vi "UI_setPlayer.vi"(7 "action":enum16{"set refs", "set player", "next player"}(ring)=enum."next player", 8 "error in (no error)":errorcluster, 9 "player":enum16{"one", "two", "three"}(ring), 11 "LED refs":refnum<vi>[](array[refnum])) -> (0 "error out":errorcluster, 2 "Player":i32)   [LabVIEW 2020]
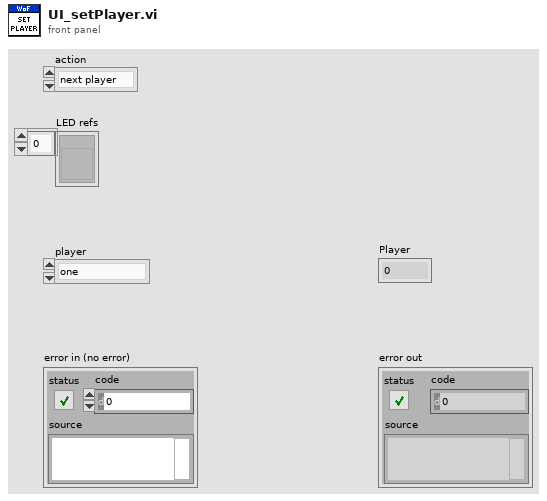
[diagram p1: front panel]
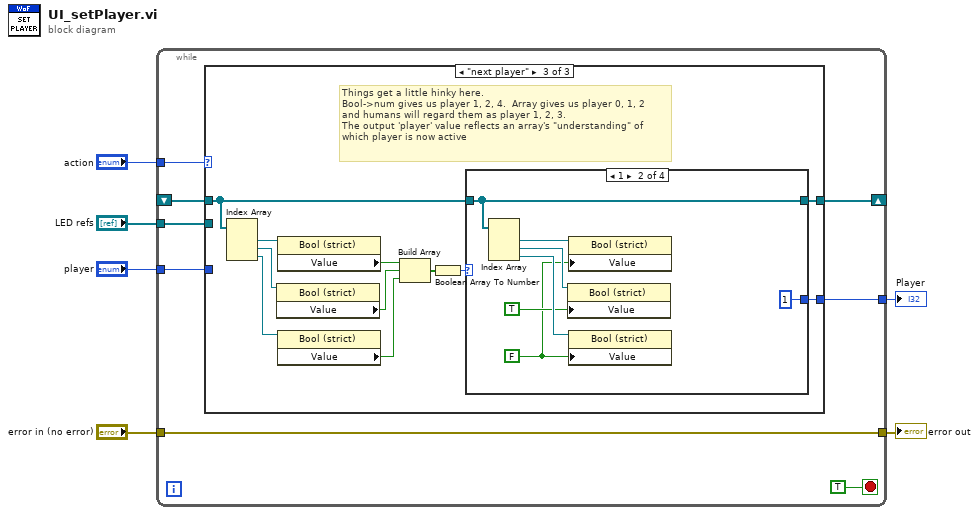
[diagram p0: block diagram]
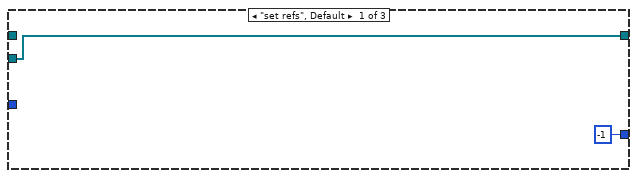
[diagram p2: hidden frame]
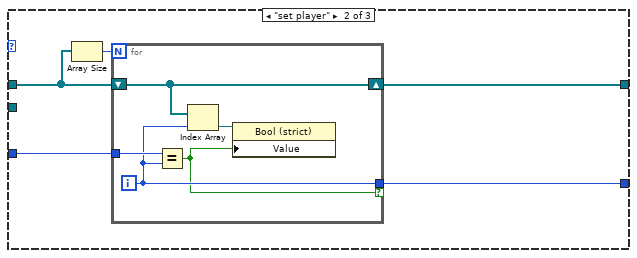
[diagram p3: hidden frame]
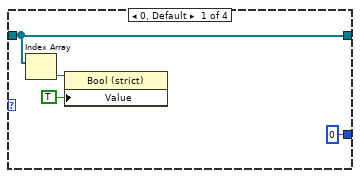
[diagram p4: hidden frame]
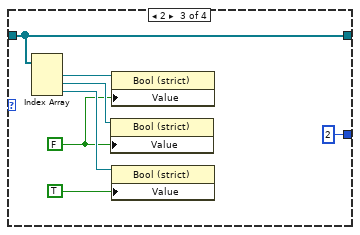
[diagram p5: hidden frame]
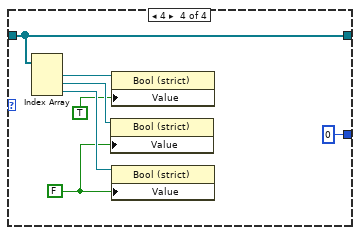
[diagram p6: hidden frame]
diagram:
  n1 = while {
    tunnel: "action" -> [w14]
    tunnel: "player" -> [w13]
    tunnel: "LED refs" -> [w11]
    shift-right: [w10] -> _
    shift-left: _ -> [w9]
    tunnel: [w8] -> w3
    tunnel: "error in (no error)" -> [w7]
    tunnel: [w7] -> w1
    stop <- TRUE stop-if-true
    n2 = case shown="\"next player\"" w14 {
      tunnel: w13 -> [_ w20 _]
      tunnel: w11 -> [w16 _ _]
      tunnel: [w16 w21 w28] -> w10
      tunnel: w9 -> [_ w18 w30]
      tunnel: [-1 w19 w27] -> w8
      frame "set refs", Default {
      }
      frame "set player" {
        n3 = Array Size(array=w18) -> (size(s)=w17:i32)
        n4 = for {
          N: w17 -> [_]
          shift-right: [w26] -> w21
          shift-left: w18 -> [w26]
          tunnel: w20 -> [w25]
          tunnel: [w24] -> w19 if=w22
          i -> [w24]
          n5 = Equal?(x=w25, y=w24) -> (x = y?=w22:bool)
          n6 = Index Array(array=w26, index=w24) -> (element=w23:refnum<vi>)
          n7 = property class="Bool (strict)"(reference=w23, "Value"=w22) -> ()  [unwired: 1 in, 2 out]
        }
      }
      frame "next player" {
        # "Things get a little hinky here.\nBool->num gives us player 1, 2, 4.  Array gives us player 0, 1, 2\nand humans will regard them as player 1, 2, 3.\nThe output 'player' value reflects an array's \"understanding\" of\nwhich player is now active"
        n8 = Index Array(array=w30) -> (element #1=w37:refnum<vi>, element #2=w36:refnum<vi>, element #3=w35:refnum<vi>)  [unwired: 3 in]
        n9 = property class="Bool (strict)"(reference=w36) -> ("Value"=w33:bool)  [unwired: 1 in, 2 out]
        n10 = property class="Bool (strict)"(reference=w37) -> ("Value"=w34:bool)  [unwired: 1 in, 2 out]
        n11 = property class="Bool (strict)"(reference=w35) -> ("Value"=w32:bool)  [unwired: 1 in, 2 out]
        n12 = Build Array(w34, w33, w32) -> (w31:bool[])
        n13 = Boolean Array To Number(Boolean array=w31) -> (number=w29:u32)
        n14 = case shown="1" w29 {
          tunnel: w30 -> [w41 w45 w52 w59]
          tunnel: [w41 w45 w52 w59] -> w28
          tunnel: [0 1 2 0] -> w27
          frame 0, Default {
            n15 = Index Array(array=w41) -> (element=w40:refnum<vi>)  [unwired: 1 in]
            n16 = property class="Bool (strict)"(reference=w40, "Value"=TRUE) -> ()  [unwired: 1 in, 2 out]
          }
          frame 1 {
            w43 = FALSE
            n17 = Index Array(array=w45) -> (element #1=w46:refnum<vi>, element #2=w47:refnum<vi>, element #3=w48:refnum<vi>)  [unwired: 3 in]
            n18 = property class="Bool (strict)"(reference=w47, "Value"=TRUE) -> ()  [unwired: 1 in, 2 out]
            n19 = property class="Bool (strict)"(reference=w46, "Value"=w43) -> ()  [unwired: 1 in, 2 out]
            n20 = property class="Bool (strict)"(reference=w48, "Value"=w43) -> ()  [unwired: 1 in, 2 out]
          }
          frame 2 {
            w50 = FALSE
            n21 = Index Array(array=w52) -> (element #1=w53:refnum<vi>, element #2=w54:refnum<vi>, element #3=w55:refnum<vi>)  [unwired: 3 in]
            n22 = property class="Bool (strict)"(reference=w54, "Value"=w50) -> ()  [unwired: 1 in, 2 out]
            n23 = property class="Bool (strict)"(reference=w53, "Value"=w50) -> ()  [unwired: 1 in, 2 out]
            n24 = property class="Bool (strict)"(reference=w55, "Value"=TRUE) -> ()  [unwired: 1 in, 2 out]
          }
          frame 4 {
            w58 = FALSE
            n25 = Index Array(array=w59) -> (element #1=w60:refnum<vi>, element #2=w61:refnum<vi>, element #3=w62:refnum<vi>)  [unwired: 3 in]
            n26 = property class="Bool (strict)"(reference=w61, "Value"=w58) -> ()  [unwired: 1 in, 2 out]
            n27 = property class="Bool (strict)"(reference=w60, "Value"=TRUE) -> ()  [unwired: 1 in, 2 out]
            n28 = property class="Bool (strict)"(reference=w62, "Value"=w58) -> ()  [unwired: 1 in, 2 out]
          }
        }
      }
    }
  }
  "Player" <- w3
  "error out" <- w1
